vi "InitializeDirectoryMetadata.vi"(8 "Error in":errorcluster, 9 "Path":path, 10 "Type":string, 11 "ID":string) -> (0 "Error out":errorcluster, 3 "DirectoryMetadata instance":refnum<data-value>)   [LabVIEW 2017, in "DirectoryMetadata.lvclass"]
uses:
  DirectoryMetadata.lvclass
  DirectoryMetadata.lvclass/DirectoryMetadata.ctl
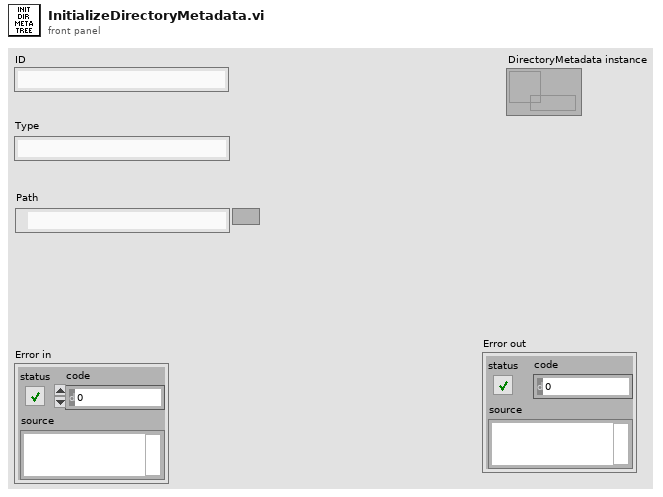
[diagram p1: front panel]
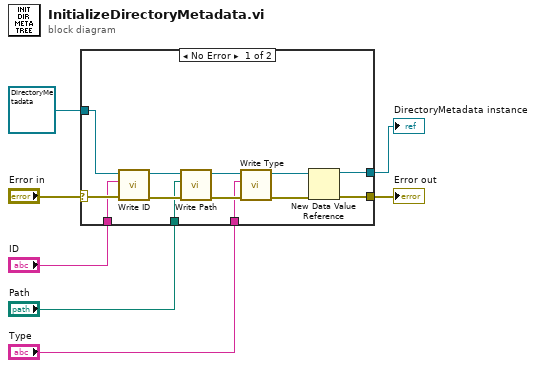
[diagram p0: block diagram]
diagram:
  n1 = case shown="No Error" "Error in" {
    selector: "Error in" -> [w18 w21]
    tunnel: [w20 w21] -> w4
    tunnel: refnum<class "DirectoryMetadata.lvclass"> refnum ("ClassMetadata.lvclass") -> [w17 _]
    tunnel: [w19 _] -> w6
    tunnel: "Type" -> [w10 _]
    tunnel: "Path" -> [w9 _]
    tunnel: "ID" -> [w8 _]
    frame No Error {
      n2 = call "Write ID.vi"("error in (no error)"=w18, "ID"=w8, "ClassMetadata in"=w17) -> ("error out"=w16:errorcluster, "ClassMetadata out"=w15:refnum<class "DirectoryMetadata.lvclass">)  [unwired: 7 in]
      n3 = call "Write Path.vi"("error in (no error)"=w16, "Path"=w9, "ClassMetadata in"=w15) -> ("error out"=w14:errorcluster, "ClassMetadata out"=w11:refnum<class "DirectoryMetadata.lvclass">)  [unwired: 7 in]
      n4 = call "Write Type.vi"("error in (no error)"=w14, "Type"=w10, "ClassMetadata in"=w11) -> ("error out"=w13:errorcluster, "ClassMetadata out"=w12:refnum<class "DirectoryMetadata.lvclass">)  [unwired: 7 in]
      n5 = New Data Value Reference(data value=w12, error in=w13) -> (data value reference=w19:refnum<data-value>, error out=w20:errorcluster)
    }
    frame Error {
    }
  }
  "DirectoryMetadata instance" <- w6
  "Error out" <- w4
